vi "PROG 2 - Conversion of Temperatures Using Fomula.vi"() -> ()   [LabVIEW 2012]
uses:
  conversion between two temperatures.ctl
  <vilib>/express/express arith-compare/Formula/XNode/ExpressFormulaBlockNode.xnode
panel:
  out "Temperature in Degree Celsius Scale":dbl
  in  "Temperature in Degree Fahrenheit  Scale":dbl
  out "Thermometer (Degree Celsius)":dbl(slide) scale=0.0..100.0
  out "Thermometer (Fahrenheit)":T1 scale=0.0..100.0
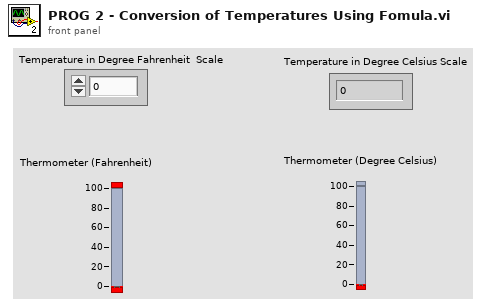
[diagram p1: front panel]
types:
  T1 = typedef "conversion between two temperatures.ctl" = dbl
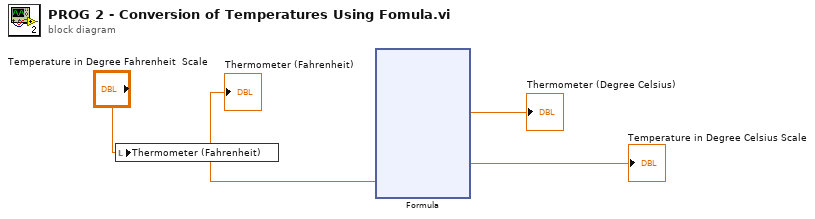
[diagram p0: block diagram]
diagram:
  n1 = local write "Thermometer (Fahrenheit)"("Temperature in Degree Fahrenheit  Scale") -> ()
  n2 = xnode "Formula"("X2"="Temperature in Degree Fahrenheit  Scale") -> ("Result"=→"Thermometer (Degree Celsius)" →"Temperature in Degree Celsius Scale":dbl)  [unwired: 2 in, 1 out]
  "Thermometer (Fahrenheit)" <- "Temperature in Degree Fahrenheit  Scale"
